vi "Constructor.vi"(6 "Precision":u8, 7 "ComparisonType":T1, 8 "error in":errorcluster, 9 "HigherBond":dbl, 10 "LowerBound":dbl, 11 "Name":string) -> (0 "error out":errorcluster, 3 "RealMeasureLimit":refnum<class "RealMeasureLimit.lvclass">)   [LabVIEW 2021, in "ProligentXMLGenerator.lvlib" / "RealMeasureLimit.lvclass"]
uses:
  RealMeasureLimit.lvclass
  RealMeasureLimit.lvclass/RealMeasureLimit.ctl
  MeasureLimit/MeasureLimit.lvclass
  Data.ctl
  RangeMeasureLimit/RangeMeasureLimit.lvclass
  Base/Decimal/Decimal.lvclass
  C:/Projects/proligent-xml-generator-labview/src/ProligentXMLGenerator/Measure/RangeMeasureLimit/RangeMeasureLimit.lvclass
  C:/Projects/proligent-xml-generator-labview/src/ProligentXMLGenerator/Measure/MeasureLimit/MeasureLimit.lvclass
  RangeMeasureLimit/ComparisonType.ctl
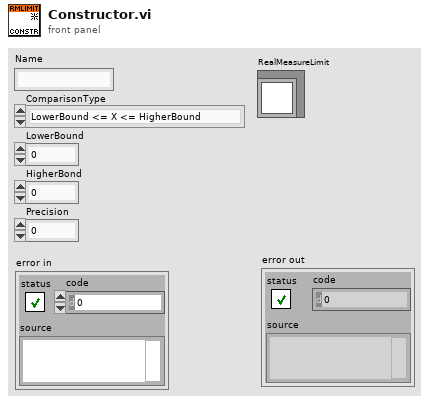
[diagram p1: front panel]
types:
  T1 = typedef "ProligentXMLGenerator.lvlib/RangeMeasureLimit.lvclass/ComparisonType.ctl" = enum16{"LowerBound <= X <= HigherBound", "LowerBound < X <= HigherBound", "LowerBound <= X < HigherBound", "LowerBound < X < HigherBound", "LowerBound <= X", "LowerBound < X", "X <= HigherBound", "X < HigherBound", "X == HigherBound", "X != HigherBound", "X <= LowerBound OR HigherBound <= X", "X < LowerBound OR HigherBound <= X", "X <= LowerBound OR HigherBound < X", "X < LowerBound OR HigherBound < X"}
  T2 = typedef "ProligentXMLGenerator.lvlib/RealMeasureLimit.lvclass/Data.ctl" = cluster{"LowerBound":refnum<class "Decimal.lvclass">, "HigherBound":refnum<class "Decimal.lvclass">}
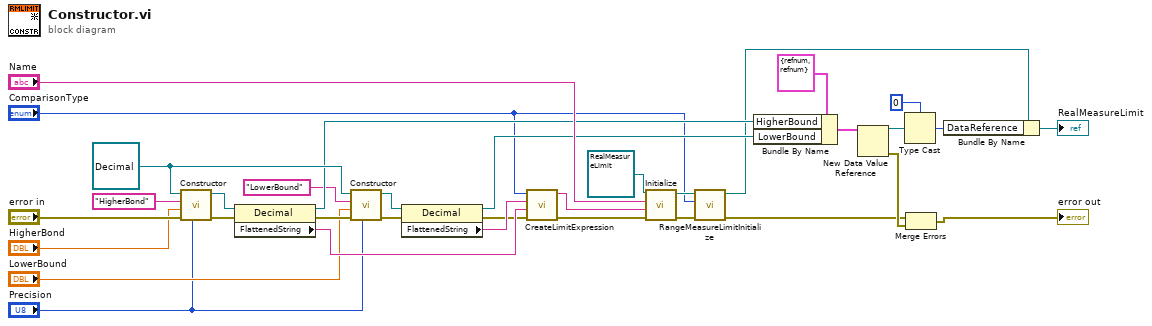
[diagram p0: block diagram]
diagram:
  w20 = refnum<class "Decimal.lvclass"> refnum ("ProligentResultProcessor:Decimal")
  n1 = call-dynamic "Constructor.vi"("Precision"="Precision", "error in"="error in", "Value"="HigherBond", "Name"="HigherBond", "Decimal in"=w20) -> ("error out"=w21:errorcluster, "Decimal out"=w16:refnum<class "Decimal.lvclass">)  [unwired: 5 in]
  n2 = property class="Decimal"(reference=w16, error in=w21) -> (reference out=w8:refnum<class "Decimal.lvclass">, error out=w17:errorcluster, "FlattenedString"=w15:string)
  n3 = call-dynamic "Constructor.vi"("Precision"="Precision", "error in"=w17, "Value"="LowerBound", "Name"="LowerBound", "Decimal in"=w20) -> ("error out"=w12:errorcluster, "Decimal out"=w13:refnum<class "Decimal.lvclass">)  [unwired: 5 in]
  n4 = property class="Decimal"(reference=w13, error in=w12) -> (reference out=w9:refnum<class "Decimal.lvclass">, error out=w10:errorcluster, "FlattenedString"=w11:string)
  n5 = call "CreateLimitExpression.vi"("error in"=w10, "HigherBound"=w15, "LowerBound"=w11, "ComparisonType"="ComparisonType") -> ("error out"=w24:errorcluster, "LimitExpression"=w23:string)  [unwired: 6 in]
  n6 = call "Initialize.vi"("error in"=w24, "LimitExpression"=w23, "Name"="Name", "MeasureLimit in"=refnum<class "RealMeasureLimit.lvclass"> refnum ("ProligentResultProcessor:RealMeasureLimit.lvclass")) -> ("error out"=w3:errorcluster, "MeasureLimit out"=w5:refnum<class "RealMeasureLimit.lvclass">)  [unwired: 6 in]
  n7 = call "RangeMeasureLimitInitialize.vi"("error in"=w3, "ComparisonType"="ComparisonType", "RangeMeasureLimit in"=w5) -> ("error out"=w2:errorcluster, "RangeMeasureLimit out"=w4:refnum<class "RealMeasureLimit.lvclass">)  [unwired: 7 in]
  n8 = Bundle By Name(cluster=T2 {"LowerBound"=refnum, "HigherBound"=refnum} ("Data"), "HigherBound"=w8, "LowerBound"=w9) -> (w30:T2)
  n9 = New Data Value Reference(data value=w30) -> (data value reference=w31:refnum<data-value>, error out=w34:errorcluster)  [unwired: 1 in]
  n10 = Type Cast(type=u64 0, x=w31) -> (*(type *) &x=w33:u64)
  n11 = Merge Errors(w2, w34) -> (→"error out":errorcluster)
  n12 = Bundle By Name(cluster=w4, "DataReference"=w33) -> (→"RealMeasureLimit":refnum<class "RealMeasureLimit.lvclass">)
